vi "Prepare Service Request.vi"(8 "error in (no error)":errorcluster, 10 "Status Register":T1={"Parameter Changed from front panel"=FALSE, "Data Ready"=FALSE, "Scan Finished"=TRUE, "Counter Overrun"=FALSE, "Rate Error"=FALSE, "Recall Error"=FALSE, "Service Request"=FALSE, "Command Error"=FALSE}, 11 "VISA resource name":refnum<visa-resource-name>) -> (0 "error out":errorcluster, 3 "VISA resource name out":refnum<visa-resource-name>)   [LabVIEW 2015, in "SR400.lvlib"]
doc: "Default request: tell when \"scan finished\" is true."
uses:
  SR400.lvlib
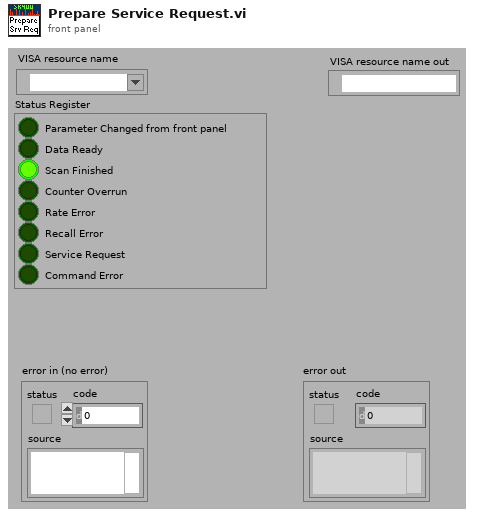
[diagram p1: front panel]
types:
  T1 = cluster{"Parameter Changed from front panel":bool, "Data Ready":bool, "Scan Finished":bool, "Counter Overrun":bool, "Rate Error":bool, "Recall Error":bool, "Service Request":bool, "Command Error":bool}
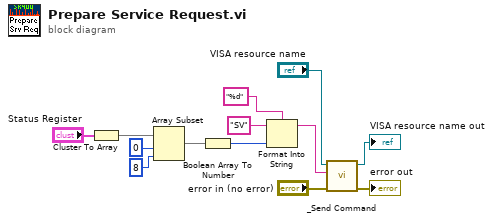
[diagram p0: block diagram]
diagram:
  n1 = Cluster To Array(cluster="Status Register") -> (array=w10:bool[])
  n2 = Array Subset(array=w10, index=0, length=8) -> (w9:bool[])
  n3 = Boolean Array To Number(Boolean array=w9) -> (number=w2:u32)
  n4 = Format Into String(format string="%d", initial string="SV", w2) -> (resulting string=w1:string)  [unwired: 1 in, 1 out]
  n5 = call "_Send Command.vi"("error in (no error)"="error in (no error)", "Command"=w1, "VISA resource name"="VISA resource name") -> ("error out"=→"error out":errorcluster, "VISA resource name out"=→"VISA resource name out":refnum<visa-resource-name>)  [unwired: 1 in, 6 out]
